vi "specu1a 1.0.0 Set EEPROM default.vi"(0 "Device Handle":i32, 3 "error in (no error)":errorcluster) -> (5 "Device Handle out":i32, 7 "error out":errorcluster)   [LabVIEW 2010]
uses:
  Controls/specu1a 1.0.0 EEPROM default mode.ctl
  SpecUSB Drivers/DLL&Driver/specu1a.dll
panel:
  out "Default mode 2":T1
  in  "Default mode":T1
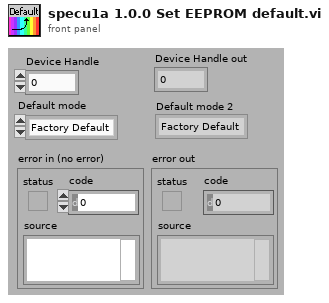
[diagram p1: front panel]
types:
  T1 = typedef "specu1a 1.0.0 EEPROM default mode.ctl" = enum8{"Factory Default", "Current", "No Change"}
  T2 = typedef "specu1a 1.0.0 Error codes.ctl" = enum16{"INVALID_HANDLE_VALUE", "USBDEV_SUCCESS", "USBDEV_INVALID_HANDLE", "USBDEV_UNSUCCESS", "USBDEV_INVALID_VALUE", "USBDEV_CHECK_NORMAL", "USBDEV_CHECK_INVALID", "USBDEV_CHECK_REMOVE", "USBDEV_CHECK_OTHER", "USBDEV_RESET_ERROR", "USBDEV_BULKSIZE_ERROR", "USBDEV_BULK_READ_ERROR", "USBDEV_BULK_NOT_UPDATED", "USBDEV_TIME_OVER_ERROR", "USBDEV_TIME_UNDER_ERROR", "USBDEV_TIME_SET_ERROR", "USBDEV_SET_GAIN_ERROR", "USBDEV_GET_TEMP_ERROR", "USBDEV_SET_TRIGGER_ERROR", "USBDEV_RW_EEP_ADDR_ERROR", "USBDEV_RW_EEP_SIZE_ERROR", "USBDEV_RW_EEP_OVER_ERROR", "USBDEV_RW_EEP_ERROR", "UNITID_PRODUCTID_CONFLICT", "UNKNOWN_ERROR"}
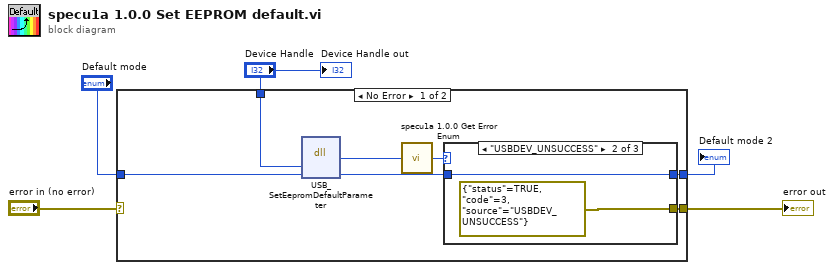
[diagram p0: block diagram]
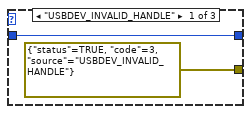
[diagram p2: hidden frame]
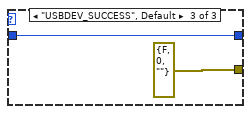
[diagram p3: hidden frame]
diagram:
  n1 = case shown="No Error" "error in (no error)" {
    selector: "error in (no error)" -> [_ w20]
    tunnel: [w11 w20] -> w4
    tunnel: "Device Handle" -> [w9 _]
    tunnel: [w10 w19] -> w2
    tunnel: "Default mode" -> [w7 w19]
    frame No Error {
      n2 = dll-call lib="C:/SpecUSB Drivers/DLL&Driver/specu1a.dll" fn="USB_SetEepromDefaultParameter" label="1.0.0 Set default EEPROM"("Device Handle"=w9, "Mode"=w7) -> (w8:u16, "Mode"=w6:u8)  [unwired: 4 in, 2 out]
      n3 = call "specu1a 1.0.0 Get Error Enum.vi"("Error Code in"=w8) -> ("Specu1a 1.0.0 Error code out"=w12:T2)  [unwired: 4 in]
      n4 = case shown="\"USBDEV_UNSUCCESS\"" w12 {
        tunnel: [w13 w15 w17] -> w10
        tunnel: [errorcluster {"status"=TRUE, "code"=3, "source"="USBDEV_INVALID_HANDLE"} ("error out") errorcluster {"status"=TRUE, "code"=3, "source"="USBDEV_UNSUCCESS"} ("error out") errorcluster {"status"=FALSE, "code"=0, "source"=""} ("error out")] -> w11
        tunnel: w6 -> [w13 w15 w17]
        frame "USBDEV_INVALID_HANDLE" {
        }
        frame "USBDEV_UNSUCCESS" {
        }
        frame "USBDEV_SUCCESS", Default {
        }
      }
    }
    frame Error {
    }
  }
  "error out" <- w4
  "Default mode 2" <- w2
  "Device Handle out" <- "Device Handle"
